vi "Init.vi"(8 "error in (no error)":errorcluster, 11 "GameObject in":refnum<class "GameObject.lvclass">) -> (0 "error out":errorcluster, 3 "GameObject out":refnum<class "GameObject.lvclass">)   [LabVIEW 2019, in "RT_Game.lvlib" / "GameObject.lvclass"]
uses:
  GameObject.lvclass
  GameObject.lvclass/GameObject.ctl
  Write Collides_.vi
  Write ManualVelocity.vi
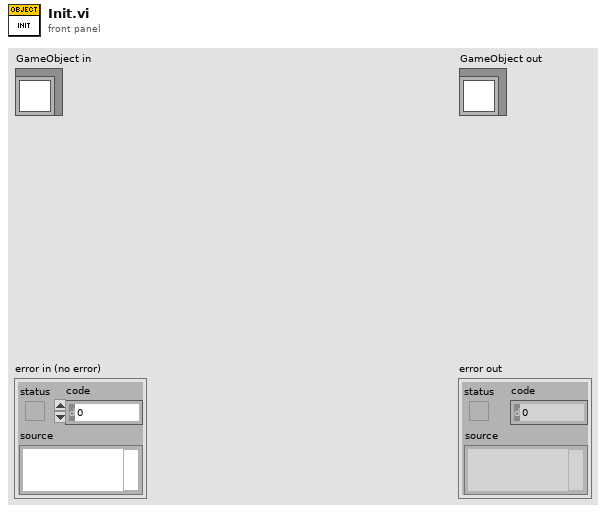
[diagram p1: front panel]
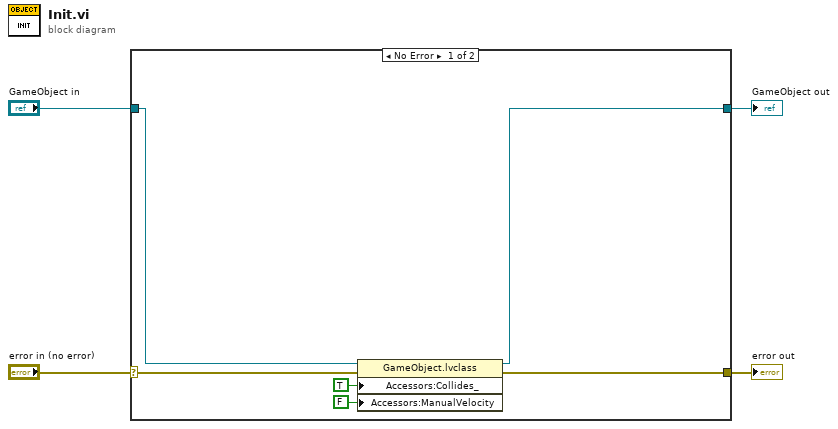
[diagram p0: block diagram]
diagram:
  n1 = case shown="No Error" "error in (no error)" {
    selector: "error in (no error)" -> [w10 w12]
    tunnel: [w9 w12] -> w3
    tunnel: [w7 w11] -> w1
    tunnel: "GameObject in" -> [w8 w11]
    frame No Error {
      n2 = property class="GameObject.lvclass"(reference=w8, error in=w10, "Accessors:Collides_"=TRUE ("Collides_"), "Accessors:ManualVelocity"=FALSE ("ManualVelocity")) -> (reference out=w7:refnum<class "GameObject.lvclass">, error out=w9:errorcluster)
    }
    frame Error {
    }
  }
  "error out" <- w3
  "GameObject out" <- w1
